vi "BinSearchVIHotwarm.vi"(8 "X0":sgl=0.5, 11 "Ring":i16(ring) items=["Warm", "Cold"]) -> (3 "Xpot":sgl)   [LabVIEW 2019]
uses:
  <vilib>/Platform/TimedLoop/XDataNode/timing_clust.ctl
  <vilib>/Platform/TimedLoop/XDataNode/nitl_modes.ctl
  <vilib>/Platform/TimedLoop/XDataNode/wakeup.ctl
  <vilib>/rvi/Emulation/niFpgaGetClockAttributes.vi
  <vilib>/rvi/Emulation/niFpgaSctlEmulationGetInTimedLoop.vi
  <vilib>/rvi/Emulation/niFpgaEmulationReportErrorSimple.vi
  <vilib>/rvi/Emulation/niFpgaCriticalErrorInLSC.vi
  <vilib>/Platform/TimedLoop/XDataNode/XDataNode.xnode
  <vilib>/Platform/TimedLoop/XDataNode/XDNodeRunTimeDep.lvlib
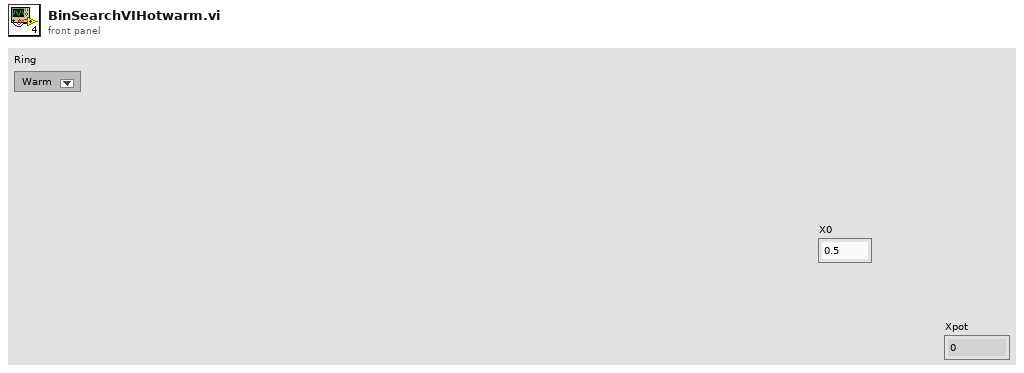
[diagram p1: front panel]
types:
  T1 = typedef "XDNodeRunTimeDep.lvlib/timing_clust.ctl" = cluster{"Expected End [f-1]":u64, "Actual End [f-1]":u64, "Finished Late? [f-1]":bool, "Expected End [i-1]":u64, "Actual End [i-1]":u64, "Finished Late? [i-1]":bool, "Expected Start [i]":u64, "Actual Start [i]":u64, "Expected Start [f]":u64, "Actual Start [f]":u64, "Source Name":string, "Structure Name":string, "Period":i64, "Deadline":i64, "Offset":i64, "Start":i64, "Priority":i32, "Timeout":i32, "Mode":T2, "Wakeup Reason":T3, "Error":errorcluster, "Source Type":string, "Secondary Source Type":string, "Global End Time":u64, "Global Start Time":u64, "Frame Duration":u64, "Iteration Duration":u64, "Assigned CPU":i32, "I/O Scan Engine Mode":u32}
  T2 = typedef "XDNodeRunTimeDep.lvlib/nitl_modes.ctl" = enum32{"No Change", "Process missed periods, maintain original phase", "Discard missed periods, maintain original phase", "Process missed periods, ignore original phase", "Discard missed periods, ignore original phase"}
  T3 = typedef "XDNodeRunTimeDep.lvlib/wakeup.ctl" = enum32{"Normal", "Aborted", "Asynchronous wakeup", "Timing source error", "Timed loop error", "Timeout"}
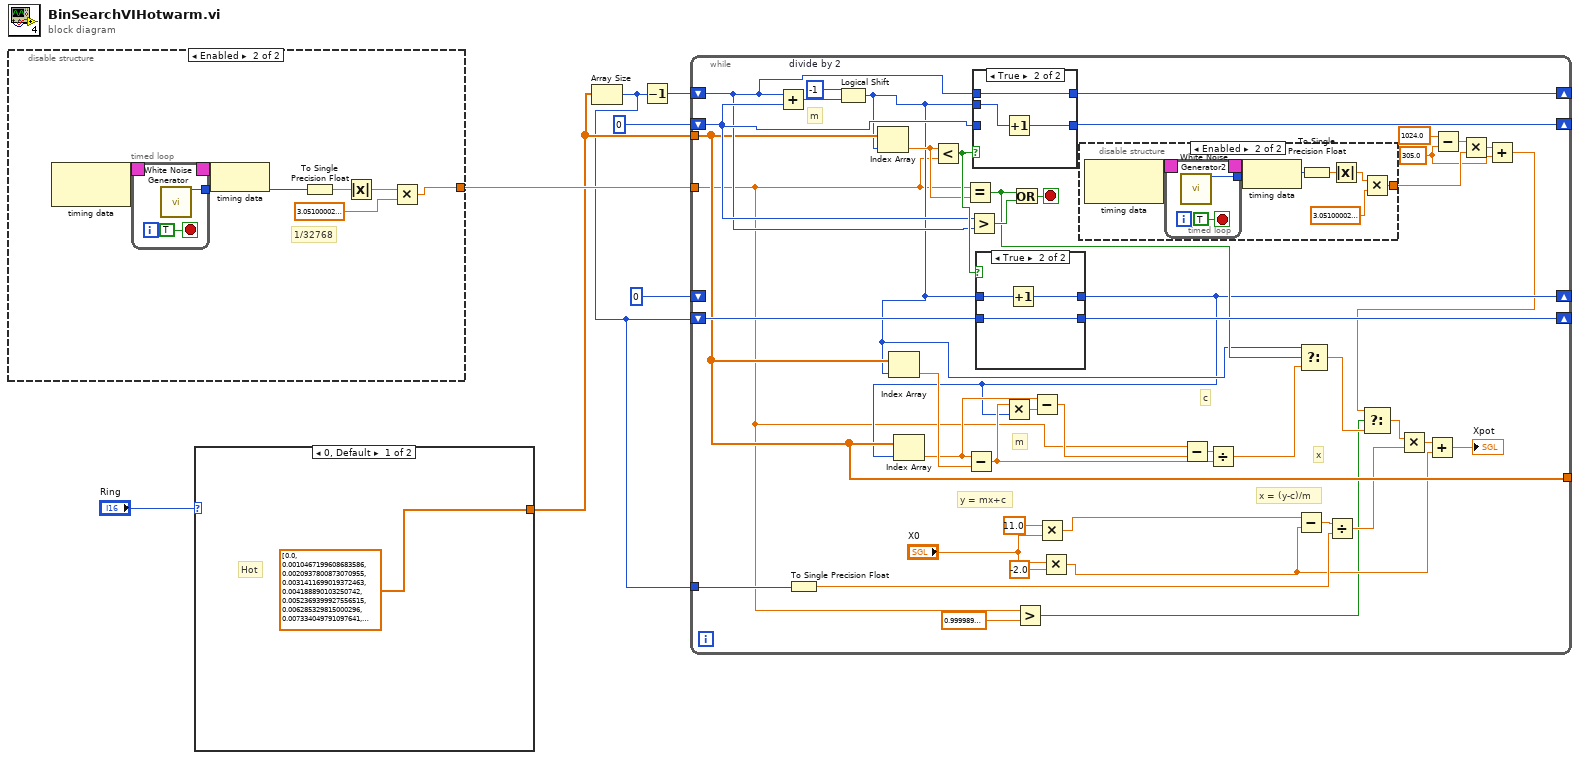
[diagram p0: block diagram]
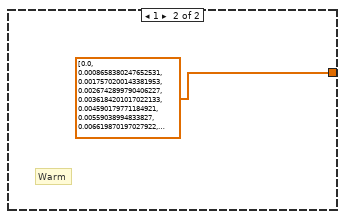
[diagram p2: hidden frame]
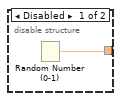
[diagram p3: hidden frame]
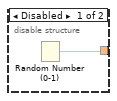
[diagram p4: hidden frame]
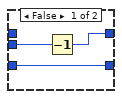
[diagram p6: hidden frame]
diagram:
  n1 = disable-structure shown="Enabled" {
    disable-tunnel: [w8 w11] -> w4
    frame Disabled {
      n2 = Random Number (0-1)() -> (number: 0 to 1=w8:dbl)
    }
    frame Enabled {
      # "1/32768"
      n3 = node-c288() -> (w10:T1)  [unwired: 1 in]
      n4 = timed-loop {
        timing: w10 -> [_]
        timing-out: [_] -> w9
        tunnel: [w17] -> w15
        stop <- TRUE stop-if-true
        n5 = call "White Noise Generator"() -> ("white noise out"=w17:i16)  [unwired: 15 in]
      }
      n6 = node-c288(w9) -> ()
      n7 = To Single Precision Float(number=w15) -> (single precision float=w13:sgl)
      n8 = Absolute Value(x=w13) -> (abs(x)=w12:sgl)
      n9 = Multiply(x=w12, y=sgl 3.051e-05) -> (x*y=w11:sgl)
    }
  }
  n10 = case shown="0, Default" "Ring" {
    tunnel: [sgl[] [0.0, 0.00104672, 0.00209378, 0.00314117, 0.00418889, 0.00523694, 0.00628533, 0.00733405, 0.0083831, 0.00943249, 0.0104822, 0.0115323, 0.0125826, 0.0136334, 0.0146844, 0.0157358, 0.0167875, 0.0178396, 0.018892, 0.0199447, 0.0209977, 0.0220511, 0.0231048, 0.0241589, 0.0252133, 0.026268, 0.0273231, 0.0283785, 0.0294342, 0.0304902, 0.0315466, 0.0326032, 0.0336601, 0.0347173, 0.0357748, 0.0368325, 0.0378905, 0.0389487, 0.0400072, 0.0410658, 0.0421247, 0.0431839, 0.0442432, 0.0453027, 0.0463624, 0.0474222, 0.0484823, 0.0495425, 0.0506029, 0.0516634, 0.0527241, 0.0537849, 0.0548458, 0.0559069, 0.0569681, 0.0580294, 0.0590909, 0.0601524, 0.061214, 0.0622757, 0.0633376, 0.0643995, 0.0654614, 0.0665235, 0.0675856, 0.0686478, 0.0697101, 0.0707724, 0.0718348, 0.0728972, 0.0739596, 0.0750221, 0.0760847, 0.0771473, 0.0782099, 0.0792725, 0.0803352, 0.0813978, 0.0824605, 0.0835233, 0.084586, 0.0856487, 0.0867115, 0.0877742, 0.088837, 0.0898997, 0.0909625, 0.0920252, 0.093088, 0.0941507, 0.0952134, 0.0962761, 0.0973388, 0.0984015, 0.0994642, 0.100527, 0.10159, 0.102652, 0.103715, 0.104777, 0.10584, 0.106902, 0.107965, 0.109027, 0.11009, 0.111152, 0.112215, 0.113277, 0.114339, 0.115402, 0.116464, 0.117526, 0.118589, 0.119651, 0.120713, 0.121775, 0.122837, 0.123899, 0.124961, 0.126023, 0.127085, 0.128147, 0.129209, 0.130271, 0.131333, 0.132395, 0.133457, 0.134519, 0.135581, 0.136642, 0.137704, 0.138766, 0.139828, 0.140889, 0.141951, 0.143013, 0.144075, 0.145136, 0.146198, 0.14726, 0.148321, 0.149383, 0.150444, 0.151506, 0.152568, 0.153629, 0.154691, 0.155752, 0.156814, 0.157876, 0.158937, 0.159999, 0.16106, 0.162122, 0.163184, 0.164245, 0.165307, 0.166368, 0.16743, 0.168492, 0.169553, 0.170615, 0.171677, 0.172739, 0.1738, 0.174862, 0.175924, 0.176986, 0.178048, 0.17911, 0.180171, 0.181233, 0.182295, 0.183357, 0.184419, 0.185482, 0.186544, 0.187606, 0.188668, 0.18973, 0.190792, 0.191855, 0.192917, 0.19398, 0.195042, 0.196104, 0.197167, 0.19823, 0.199292, 0.200355, 0.201418, 0.20248, 0.203543, 0.204606, 0.205669, 0.206732, 0.207795, 0.208858, 0.209921, 0.210985, 0.212048, 0.213111, 0.214174, 0.215238, 0.216301, 0.217365, 0.218428, 0.219492, 0.220556, 0.22162, 0.222683, 0.223747, 0.224811, 0.225875, 0.226939, 0.228003, 0.229067, 0.230131, 0.231196, 0.23226, 0.233324, 0.234389, 0.235453, 0.236517, 0.237582, 0.238646, 0.239711, 0.240776, 0.24184, 0.242905, 0.24397, 0.245034, 0.246099, 0.247164, 0.248229, 0.249293, 0.250358, 0.251423, 0.252488, 0.253553, 0.254618, 0.255683, 0.256747, 0.257812, 0.258877, 0.259942, 0.261007, 0.262072, 0.263136, 0.264201, 0.265266, 0.266331, 0.267395, 0.26846, 0.269525, 0.270589, 0.271654, 0.272718, 0.273782, 0.274847, 0.275911, 0.276975, 0.278039, 0.279103, 0.280167, 0.28123, 0.282294, 0.283357, 0.284421, 0.285484, 0.286547, 0.28761, 0.288673, 0.289735, 0.290798, 0.29186, 0.292922, 0.293984, 0.295046, 0.296107, 0.297169, 0.29823, 0.29929, 0.300351, 0.301411, 0.302471, 0.303531, 0.304591, 0.30565, 0.306709, 0.307768, 0.308826, 0.309884, 0.310942, 0.311999, 0.313056, 0.314112, 0.315169, 0.316225, 0.31728, 0.318336, 0.319391, 0.320445, 0.3215, 0.322554, 0.323607, 0.32466, 0.325713, 0.326766, 0.327818, 0.32887, 0.329922, 0.330973, 0.332024, 0.333075, 0.334125, 0.335175, 0.336225, 0.337274, 0.338323, 0.339372, 0.34042, 0.341468, 0.342515, 0.343563, 0.34461, 0.345656, 0.346703, 0.347749, 0.348794, 0.34984, 0.350884, 0.351929, 0.352973, 0.354017, 0.355061, 0.356104, 0.357147, 0.35819, 0.359232, 0.360274, 0.361316, 0.362357, 0.363398, 0.364439, 0.365479, 0.366519, 0.367559, 0.368598, 0.369637, 0.370676, 0.371714, 0.372752, 0.37379, 0.374828, 0.375865, 0.376901, 0.377938, 0.378974, 0.380009, 0.381045, 0.38208, 0.383115, 0.384149, 0.385183, 0.386217, 0.38725, 0.388283, 0.389316, 0.390349, 0.391381, 0.392412, 0.393444, 0.394475, 0.395506, 0.396536, 0.397566, 0.398596, 0.399626, 0.400655, 0.401684, 0.402712, 0.40374, 0.404768, 0.405796, 0.406823, 0.40785, 0.408877, 0.409903, 0.410929, 0.411954, 0.41298, 0.414005, 0.415029, 0.416053, 0.417077, 0.418101, 0.419124, 0.420147, 0.42117, 0.422192, 0.423214, 0.424236, 0.425257, 0.426278, 0.427299, 0.428319, 0.42934, 0.430359, 0.431379, 0.432398, 0.433417, 0.434435, 0.435453, 0.436471, 0.437488, 0.438506, 0.439522, 0.440539, 0.441555, 0.442571, 0.443586, 0.444602, 0.445617, 0.446631, 0.447645, 0.448659, 0.449673, 0.450686, 0.451699, 0.452712, 0.453724, 0.454736, 0.455748, 0.456759, 0.45777, 0.458781, 0.459791, 0.460802, 0.461811, 0.462821, 0.46383, 0.464839, 0.465847, 0.466855, 0.467863, 0.468871, 0.469878, 0.470885, 0.471891, 0.472897, 0.473903, 0.474909, 0.475914, 0.476919, 0.477924, 0.478928, 0.479932, 0.480936, 0.481939, 0.482942, 0.483945, 0.484947, 0.48595, 0.486951, 0.487953, 0.488954, 0.489955, 0.490955, 0.491955, 0.492955, 0.493955, 0.494954, 0.495953, 0.496952, 0.49795, 0.498948, 0.499946, 0.500943, 0.50194, 0.502937, 0.503933, 0.504929, 0.505925, 0.50692, 0.507915, 0.50891, 0.509905, 0.510899, 0.511893, 0.512886, 0.51388, 0.514872, 0.515865, 0.516857, 0.517849, 0.518841, 0.519832, 0.520823, 0.521814, 0.522804, 0.523794, 0.524784, 0.525774, 0.526763, 0.527752, 0.52874, 0.529728, 0.530716, 0.531704, 0.532691, 0.533678, 0.534665, 0.535651, 0.536637, 0.537623, 0.538608, 0.539593, 0.540578, 0.541562, 0.542546, 0.54353, 0.544514, 0.545497, 0.54648, 0.547462, 0.548445, 0.549427, 0.550408, 0.55139, 0.552371, 0.553351, 0.554332, 0.555312, 0.556291, 0.557271, 0.55825, 0.559229, 0.560207, 0.561186, 0.562164, 0.563141, 0.564118, 0.565095, 0.566072, 0.567048, 0.568024, 0.569, 0.569976, 0.570951, 0.571926, 0.5729, 0.573874, 0.574848, 0.575822, 0.576795, 0.577768, 0.57874, 0.579713, 0.580685, 0.581657, 0.582628, 0.583599, 0.58457, 0.58554, 0.586511, 0.58748, 0.58845, 0.589419, 0.590388, 0.591357, 0.592325, 0.593293, 0.594261, 0.595228, 0.596195, 0.597162, 0.598129, 0.599095, 0.600061, 0.601026, 0.601992, 0.602957, 0.603921, 0.604886, 0.60585, 0.606813, 0.607777, 0.60874, 0.609703, 0.610665, 0.611627, 0.612589, 0.613551, 0.614512, 0.615473, 0.616434, 0.617394, 0.618354, 0.619314, 0.620273, 0.621233, 0.622191, 0.62315, 0.624108, 0.625066, 0.626024, 0.626981, 0.627938, 0.628895, 0.629851, 0.630807, 0.631763, 0.632719, 0.633674, 0.634629, 0.635583, 0.636538, 0.637492, 0.638445, 0.639399, 0.640352, 0.641305, 0.642257, 0.643209, 0.644161, 0.645113, 0.646064, 0.647015, 0.647966, 0.648916, 0.649866, 0.650816, 0.651765, 0.652714, 0.653663, 0.654612, 0.65556, 0.656508, 0.657456, 0.658403, 0.65935, 0.660297, 0.661243, 0.662189, 0.663135, 0.664081, 0.665026, 0.665971, 0.666916, 0.66786, 0.668804, 0.669748, 0.670691, 0.671635, 0.672577, 0.67352, 0.674462, 0.675404, 0.676346, 0.677287, 0.678228, 0.679169, 0.680109, 0.681049, 0.681989, 0.682929, 0.683868, 0.684807, 0.685746, 0.686684, 0.687622, 0.68856, 0.689497, 0.690435, 0.691371, 0.692308, 0.693244, 0.69418, 0.695116, 0.696051, 0.696986, 0.697921, 0.698856, 0.69979, 0.700724, 0.701657, 0.702591, 0.703524, 0.704457, 0.705389, 0.706321, 0.707253, 0.708185, 0.709116, 0.710047, 0.710978, 0.711908, 0.712838, 0.713768, 0.714697, 0.715626, 0.716555, 0.717484, 0.718412, 0.71934, 0.720268, 0.721195, 0.722122, 0.723049, 0.723976, 0.724902, 0.725828, 0.726754, 0.727679, 0.728604, 0.729529, 0.730453, 0.731378, 0.732301, 0.733225, 0.734148, 0.735071, 0.735994, 0.736917, 0.737839, 0.738761, 0.739682, 0.740603, 0.741524, 0.742445, 0.743365, 0.744285, 0.745205, 0.746125, 0.747044, 0.747963, 0.748882, 0.7498, 0.750718, 0.751636, 0.752553, 0.75347, 0.754387, 0.755304, 0.75622, 0.757136, 0.758052, 0.758967, 0.759882, 0.760797, 0.761712, 0.762626, 0.76354, 0.764454, 0.765367, 0.76628, 0.767193, 0.768106, 0.769018, 0.76993, 0.770841, 0.771753, 0.772664, 0.773575, 0.774485, 0.775395, 0.776305, 0.777215, 0.778124, 0.779033, 0.779942, 0.780851, 0.781759, 0.782667, 0.783574, 0.784482, 0.785389, 0.786296, 0.787202, 0.788108, 0.789014, 0.78992, 0.790825, 0.79173, 0.792635, 0.793539, 0.794443, 0.795347, 0.796251, 0.797154, 0.798057, 0.79896, 0.799862, 0.800765, 0.801666, 0.802568, 0.803469, 0.80437, 0.805271, 0.806172, 0.807072, 0.807972, 0.808871, 0.809771, 0.81067, 0.811568, 0.812467, 0.813365, 0.814263, 0.81516, 0.816058, 0.816955, 0.817851, 0.818748, 0.819644, 0.82054, 0.821436, 0.822331, 0.823226, 0.824121, 0.825015, 0.825909, 0.826803, 0.827697, 0.82859, 0.829483, 0.830376, 0.831268, 0.832161, 0.833053, 0.833944, 0.834835, 0.835727, 0.836617, 0.837508, 0.838398, 0.839288, 0.840178, 0.841067, 0.841956, 0.842845, 0.843733, 0.844622, 0.84551, 0.846397, 0.847285, 0.848172, 0.849059, 0.849945, 0.850831, 0.851717, 0.852603, 0.853489, 0.854374, 0.855259, 0.856143, 0.857027, 0.857911, 0.858795, 0.859679, 0.860562, 0.861445, 0.862327, 0.86321, 0.864092, 0.864974, 0.865855, 0.866736, 0.867617, 0.868498, 0.869378, 0.870258, 0.871138, 0.872018, 0.872897, 0.873776, 0.874655, 0.875533, 0.876411, 0.877289, 0.878167, 0.879044, 0.879921, 0.880798, 0.881674, 0.882551, 0.883427, 0.884302, 0.885178, 0.886053, 0.886927, 0.887802, 0.888676, 0.88955, 0.890424, 0.891297, 0.892171, 0.893043, 0.893916, 0.894788, 0.89566, 0.896532, 0.897404, 0.898275, 0.899146, 0.900016, 0.900887, 0.901757, 0.902627, 0.903496, 0.904366, 0.905235, 0.906103, 0.906972, 0.90784, 0.908708, 0.909575, 0.910443, 0.91131, 0.912177, 0.913043, 0.913909, 0.914775, 0.915641, 0.916506, 0.917372, 0.918236, 0.919101, 0.919965, 0.920829, 0.921693, 0.922557, 0.92342, 0.924283, 0.925146, 0.926008, 0.92687, 0.927732, 0.928594, 0.929455, 0.930316, 0.931177, 0.932037, 0.932897, 0.933757, 0.934617, 0.935476, 0.936336, 0.937194, 0.938053, 0.938911, 0.939769, 0.940627, 0.941485, 0.942342, 0.943199, 0.944055, 0.944912, 0.945768, 0.946624, 0.947479, 0.948335, 0.94919, 0.950045, 0.950899, 0.951753, 0.952607, 0.953461, 0.954314, 0.955168, 0.95602, 0.956873, 0.957725, 0.958577, 0.959429, 0.960281, 0.961132, 0.961983, 0.962834, 0.963684, 0.964534, 0.965384, 0.966234, 0.967083, 0.967932, 0.968781, 0.96963, 0.970478, 0.971326, 0.972174, 0.973021, 0.973869, 0.974715, 0.975562, 0.976409, 0.977255, 0.978101, 0.978946, 0.979791, 0.980637, 0.981481, 0.982326, 0.98317, 0.984014, 0.984858, 0.985701, 0.986544, 0.987387, 0.98823, 0.989072, 0.989914, 0.990756, 0.991598, 0.992439, 0.99328, 0.994121, 0.994962, 0.995802, 0.996642, 0.997482, 0.998321, 0.99916, 0.999999] ("Init Data Out") sgl[] [0.0, 0.000865838, 0.00175702, 0.00267429, 0.00361842, 0.00459018, 0.00559039, 0.00661987, 0.0076795, 0.00877014, 0.00989271, 0.0110481, 0.0122374, 0.0134615, 0.0147214, 0.0160181, 0.0173529, 0.0187267, 0.0201407, 0.0215961, 0.0230942, 0.0246361, 0.0262231, 0.0278565, 0.0295378, 0.0312683, 0.0330498, 0.0348832, 0.0367683, 0.0387052, 0.0406935, 0.0427329, 0.044823, 0.0469636, 0.0491541, 0.0513939, 0.0536825, 0.0560193, 0.0584036, 0.0608346, 0.0633115, 0.0658336, 0.0683999, 0.0710095, 0.0736616, 0.076355, 0.0790889, 0.0818621, 0.0846736, 0.0875224, 0.0904072, 0.0933269, 0.0962805, 0.0992667, 0.102284, 0.105332, 0.108409, 0.111514, 0.114646, 0.117803, 0.120985, 0.12419, 0.127416, 0.130664, 0.133931, 0.137217, 0.14052, 0.143839, 0.147174, 0.150523, 0.153884, 0.157258, 0.160643, 0.164038, 0.167441, 0.170853, 0.174272, 0.177698, 0.181129, 0.184564, 0.188003, 0.191445, 0.19489, 0.198336, 0.201783, 0.20523, 0.208676, 0.212122, 0.215565, 0.219007, 0.222446, 0.225881, 0.229313, 0.232741, 0.236164, 0.239582, 0.242995, 0.246402, 0.249804, 0.253199, 0.256587, 0.259969, 0.263344, 0.266712, 0.270072, 0.273425, 0.276771, 0.280108, 0.283438, 0.286761, 0.290075, 0.293381, 0.29668, 0.29997, 0.303253, 0.306527, 0.309795, 0.313054, 0.316306, 0.31955, 0.322787, 0.326016, 0.329239, 0.332454, 0.335663, 0.338865, 0.34206, 0.34525, 0.348433, 0.351611, 0.354783, 0.35795, 0.361111, 0.364268, 0.36742, 0.370568, 0.373713, 0.376853, 0.37999, 0.383123, 0.386254, 0.389383, 0.392509, 0.395634, 0.398756, 0.401878, 0.404999, 0.408119, 0.411239, 0.414359, 0.41748, 0.420602, 0.423725, 0.426849, 0.429976, 0.433104, 0.436236, 0.43937, 0.442508, 0.44565, 0.448796, 0.451946, 0.455101, 0.458262, 0.461428, 0.4646, 0.467779, 0.470964, 0.474157, 0.477357, 0.480565, 0.483782, 0.487007, 0.490241, 0.493484, 0.496738, 0.500001, 0.503275, 0.506559, 0.509855, 0.513162, 0.516481, 0.519812, 0.523156, 0.526513, 0.529882, 0.533265, 0.536662, 0.540073, 0.543498, 0.546938, 0.550393, 0.553862, 0.557348, 0.560848, 0.564365, 0.567898, 0.571446, 0.575012, 0.578594, 0.582192, 0.585808, 0.58944, 0.59309, 0.596757, 0.600441, 0.604143, 0.607862, 0.611598, 0.615352, 0.619123, 0.622911, 0.626717, 0.630539, 0.634379, 0.638235, 0.642109, 0.645998, 0.649904, 0.653825, 0.657762, 0.661715, 0.665682, 0.669664, 0.67366, 0.67767, 0.681692, 0.685727, 0.689775, 0.693833, 0.697902, 0.701981, 0.70607, 0.710167, 0.714272, 0.718383, 0.722501, 0.726624, 0.73075, 0.73488, 0.739012, 0.743145, 0.747277, 0.751408, 0.755537, 0.759661, 0.763781, 0.767894, 0.772, 0.776096, 0.780182, 0.784256, 0.788316, 0.792362, 0.79639, 0.800401, 0.804392, 0.808362, 0.812309, 0.816232, 0.820128, 0.823996, 0.827836, 0.831643, 0.835419, 0.839159, 0.842864, 0.846531, 0.850159, 0.853745, 0.857289, 0.860789, 0.864243, 0.86765, 0.871009, 0.874317, 0.877573, 0.880777, 0.883927, 0.887021, 0.890059, 0.893039, 0.89596, 0.898821, 0.901622, 0.904361, 0.907038, 0.909651, 0.912201, 0.914687, 0.917108, 0.919465, 0.921755, 0.92398, 0.926142, 0.928243, 0.930284, 0.932267, 0.934193, 0.936065, 0.937883, 0.93965, 0.941366, 0.943034, 0.944654, 0.946228, 0.947757, 0.949243, 0.950687, 0.952089, 0.953452, 0.954776, 0.956062, 0.957312, 0.958526, 0.959705, 0.960851, 0.961965, 0.963047, 0.964098, 0.965119, 0.966111, 0.967075, 0.968011, 0.968921, 0.969805, 0.970664, 0.971498, 0.972309, 0.973096, 0.973861, 0.974605, 0.975327, 0.976029, 0.976711, 0.977373, 0.978016, 0.978642, 0.979249, 0.979839, 0.980413, 0.98097, 0.981511, 0.982037, 0.982548, 0.983044, 0.983527, 0.983995, 0.98445, 0.984893, 0.985322, 0.98574, 0.986145, 0.986539, 0.986922, 0.987294, 0.987656, 0.988007, 0.988348, 0.988679, 0.989001, 0.989314, 0.989618, 0.989913, 0.9902, 0.990479, 0.99075, 0.991013, 0.991268, 0.991517, 0.991758, 0.991992, 0.99222, 0.992441, 0.992656, 0.992865, 0.993068, 0.993265, 0.993457, 0.993643, 0.993824, 0.993999, 0.99417, 0.994336, 0.994497, 0.994654, 0.994806, 0.994953, 0.995097, 0.995236, 0.995372, 0.995504, 0.995631, 0.995756, 0.995876, 0.995994, 0.996108, 0.996218, 0.996326, 0.996431, 0.996532, 0.996631, 0.996727, 0.99682, 0.99691, 0.996998, 0.997083, 0.997166, 0.997247, 0.997325, 0.997401, 0.997475, 0.997547, 0.997617, 0.997685, 0.997751, 0.997815, 0.997877, 0.997937, 0.997996, 0.998053, 0.998108, 0.998162, 0.998214, 0.998265, 0.998314, 0.998362, 0.998409, 0.998454, 0.998498, 0.998541, 0.998583, 0.998623, 0.998662, 0.9987, 0.998737, 0.998773, 0.998808, 0.998842, 0.998875, 0.998907, 0.998938, 0.998968, 0.998998, 0.999026, 0.999054, 0.999081, 0.999107, 0.999132, 0.999157, 0.999181, 0.999204, 0.999227, 0.999249, 0.99927, 0.999291, 0.999311, 0.999331, 0.99935, 0.999369, 0.999387, 0.999404, 0.999421, 0.999438, 0.999454, 0.999469, 0.999484, 0.999499, 0.999513, 0.999527, 0.999541, 0.999554, 0.999566, 0.999579, 0.999591, 0.999602, 0.999614, 0.999625, 0.999635, 0.999646, 0.999656, 0.999666, 0.999675, 0.999684, 0.999693, 0.999702, 0.999711, 0.999719, 0.999727, 0.999735, 0.999742, 0.99975, 0.999757, 0.999764, 0.99977, 0.999777, 0.999783, 0.999789, 0.999795, 0.999801, 0.999807, 0.999812, 0.999818, 0.999823, 0.999828, 0.999833, 0.999838, 0.999842, 0.999847, 0.999851, 0.999856, 0.99986, 0.999864, 0.999867, 0.999871, 0.999875, 0.999879, 0.999882, 0.999885, 0.999889, 0.999892, 0.999895, 0.999898, 0.999901, 0.999904, 0.999906, 0.999909, 0.999912, 0.999914, 0.999917, 0.999919, 0.999921, 0.999924, 0.999926, 0.999928, 0.99993, 0.999932, 0.999934, 0.999936, 0.999938, 0.99994, 0.999941, 0.999943, 0.999945, 0.999946, 0.999948, 0.999949, 0.999951, 0.999952, 0.999954, 0.999955, 0.999956, 0.999958, 0.999959, 0.99996, 0.999961, 0.999962, 0.999963, 0.999964, 0.999965, 0.999966, 0.999967, 0.999968, 0.999969, 0.99997, 0.999971, 0.999972, 0.999973, 0.999973, 0.999974, 0.999975, 0.999976, 0.999976, 0.999977, 0.999978, 0.999978, 0.999979, 0.99998, 0.99998, 0.999981, 0.999981, 0.999982, 0.999983, 0.999983, 0.999984, 0.999984, 0.999985, 0.999985, 0.999985, 0.999986, 0.999986, 0.999987, 0.999987, 0.999988, 0.999988, 0.999988, 0.999989, 0.999989, 0.999989, 0.99999, 0.99999, 0.99999, 0.999991, 0.999991, 0.999991, 0.999991, 0.999992, 0.999992, 0.999992, 0.999992, 0.999993, 0.999993, 0.999993, 0.999993, 0.999994, 0.999994, 0.999994, 0.999994, 0.999994, 0.999994, 0.999995, 0.999995, 0.999995, 0.999995, 0.999995, 0.999996, 0.999996, 0.999996, 0.999996, 0.999996, 0.999996, 0.999996, 0.999996, 0.999997, 0.999997, 0.999997, 0.999997, 0.999997, 0.999997, 0.999997, 0.999997, 0.999997, 0.999998, 0.999998, 0.999998, 0.999998, 0.999998, 0.999998, 0.999998, 0.999998, 0.999998, 0.999998, 0.999998, 0.999998, 0.999998, 0.999998, 0.999999, 0.999999, 0.999999, 0.999999, 0.999999, 0.999999, 0.999999, 0.999999, 0.999999, 0.999999, 0.999999, 0.999999, 0.999999, 0.999999, 0.999999, 0.999999, 0.999999, 1.0, 1.0, 1.0, 1.0, 1.0, 1.0, 1.0, 1.0, 1.0, 1.0, 1.0, 1.0, 1.0, 1.0, 1.0, 1.0, 1.0, 1.0, 1.0, 1.0, 1.0, 1.0, 1.0, 1.0, 1.0, 1.0, 1.0, 1.0, 1.0, 1.0, 1.0, 1.0, 1.0, 1.0, 1.0, 1.0, 1.0, 1.0, 1.0, 1.0, 1.0, 1.0, 1.0, 1.0, 1.0, 1.0, 1.0, 1.0, 1.0, 1.0, 1.0, 1.0, 1.0, 1.0, 1.0, 1.0, 1.0, 1.0, 1.0, 1.0, 1.0, 1.0, 1.0, 1.0, 1.0, 1.0, 1.0, 1.0, 1.0, 1.0, 1.0, 1.0, 1.0, 1.0, 1.0, 1.0, 1.0, 1.0, 1.0, 1.0, 1.0, 1.0, 1.0, 1.0, 1.0, 1.0, 1.0, 1.0, 1.0, 1.0, 1.0, 1.0, 1.0, 1.0, 1.0, 1.0, 1.0, 1.0, 1.0, 1.0, 1.0, 1.0, 1.0, 1.0, 1.0, 1.0, 1.0, 1.0, 1.0, 1.0, 1.0, 1.0, 1.0, 1.0, 1.0, 1.0, 1.0, 1.0, 1.0, 1.0, 1.0, 1.0, 1.0, 1.0, 1.0, 1.0, 1.0, 1.0, 1.0, 1.0, 1.0, 1.0, 1.0, 1.0, 1.0, 1.0, 1.0, 1.0, 1.0, 1.0, 1.0, 1.0, 1.0, 1.0, 1.0, 1.0, 1.0, 1.0, 1.0, 1.0, 1.0, 1.0, 1.0, 1.0, 1.0, 1.0, 1.0, 1.0, 1.0, 1.0, 1.0, 1.0, 1.0, 1.0, 1.0, 1.0, 1.0, 1.0, 1.0, 1.0, 1.0, 1.0, 1.0, 1.0, 1.0, 1.0, 1.0, 1.0, 1.0, 1.0, 1.0, 1.0, 1.0, 1.0, 1.0, 1.0, 1.0, 1.0, 1.0, 1.0, 1.0, 1.0, 1.0, 1.0, 1.0, 1.0, 1.0, 1.0, 1.0, 1.0, 1.0, 1.0, 1.0, 1.0, 1.0, 1.0, 1.0, 1.0, 1.0, 1.0, 1.0, 1.0, 1.0, 1.0, 1.0, 1.0, 1.0, 1.0, 1.0, 1.0, 1.0, 1.0, 1.0, 1.0, 1.0, 1.0, 1.0, 1.0, 1.0, 1.0, 1.0, 1.0, 1.0, 1.0, 1.0, 1.0, 1.0, 1.0, 1.0, 1.0, 1.0, 1.0, 1.0, 1.0, 1.0, 1.0, 1.0, 1.0, 1.0, 1.0, 1.0, 1.0, 1.0, 1.0, 1.0, 1.0, 1.0, 1.0, 1.0, 1.0, 1.0, 1.0, 1.0, 1.0, 1.0, 1.0, 1.0, 1.0, 1.0, 1.0, 1.0, 1.0, 1.0, 1.0, 1.0, 1.0, 1.0, 1.0, 1.0, 1.0, 1.0, 1.0, 1.0, 1.0, 1.0, 1.0, 1.0, 1.0, 1.0, 1.0, 1.0, 1.0, 1.0, 1.0, 1.0, 1.0, 1.0, 1.0, 1.0, 1.0, 1.0, 1.0, 1.0, 1.0, 1.0, 1.0, 1.0, 1.0, 1.0, 1.0, 1.0, 1.0, 1.0, 1.0, 1.0, 1.0, 1.0, 1.0, 1.0, 1.0, 1.0, 1.0, 1.0, 1.0, 1.0, 1.0, 1.0, 1.0, 1.0, 1.0, 1.0, 1.0, 1.0, 1.0, 1.0, 1.0, 1.0, 1.0, 1.0, 1.0, 1.0, 1.0, 1.0, 1.0, 1.0, 1.0, 1.0, 1.0, 1.0, 1.0, 1.0] ("Init Data Out")] -> w2
    frame 0, Default {
      # "Hot"
    }
    frame 1 {
      # "Warm"
    }
  }
  n11 = Array Size(array=w2) -> (size(s)=w1:i32)
  n12 = Decrement(x=w1) -> (x-1=w5:i32)
  n13 = while {
    tunnel: w2 -> [w55]
    tunnel: w4 -> [w34]
    shift-right: [w67] -> _
    shift-left: w5 -> [w58]
    shift-right: [w63] -> _
    shift-left: 0 -> [w59]
    shift-right: [w46] -> _
    shift-left: 0 -> [_]
    shift-right: [w60] -> _
    shift-left: w1 -> [w61]
    tunnel: [w55] -> _
    tunnel: w1 -> [w40]
    stop <- w65 stop-if-true
    w27 = sgl 305.0 ("y")
    w68 = -1  # divide by 2
    # "x"
    # "x = (y-c)/m"
    # "c"
    # "m"
    # "y = mx+c"
    # "m"
    n14 = Add(x=w58, y=w59) -> (x+y=w64:i32)
    n15 = To Single Precision Float(number=w40) -> (single precision float=w39:sgl)
    n16 = Logical Shift(y=w68, x=w64) -> (x << y=w53:i32)
    n17 = Index Array(array=w55, index=w53) -> (element=w57:sgl)
    n18 = Index Array(array=w55, index=w53) -> (element=w56:sgl)
    n19 = Less?(x=w57, y=w34) -> (x < y?=w62:bool)
    n20 = Equal?(x=w34, y=w57) -> (x = y?=w54:bool)
    n21 = Greater?(x=w59, y=w58) -> (0:w66:bool)
    n22 = case shown="True" w62 {
      tunnel: w53 -> [w90 w93]
      tunnel: [w89 w91] -> w67
      tunnel: w59 -> [w88 _]
      tunnel: [w88 w92] -> w63
      tunnel: w58 -> [_ w91]
      frame False {
        n23 = Decrement(x=w90) -> (x-1=w89:i32)
      }
      frame True {
        n24 = Increment(x=w93) -> (x+1=w92:i32)
      }
    }
    n25 = case shown="True" w62 {
      tunnel: w53 -> [w84 w87]
      tunnel: [w83 w86] -> w46
      tunnel: w61 -> [w83 w85]
      tunnel: [w84 w85] -> w60
      frame False {
      }
      frame True {
        n26 = Increment(x=w87) -> (x+1=w86:i32)
      }
    }
    n27 = Index Array(array=w55, index=w46) -> (element=w51:sgl)
    n28 = Subtract(x=w51, y=w56) -> (x-y=w48:sgl)
    n29 = Multiply(x=w48, y=w46) -> (x*y=w52:sgl)
    n30 = Or(x=w54, y=w66) -> (x .or. y?=w65:bool)
    n31 = Greater?(x=w34, y=sgl 0.99999) -> (0:w24:bool)
    n32 = Subtract(x=w51, y=w52) -> (x-y=w50:sgl)
    n33 = Multiply(x=sgl 11.0, y="X0") -> (x*y=w43:sgl)
    n34 = Multiply(x="X0", y=sgl -2.0) -> (x*y=w37:sgl)
    n35 = disable-structure shown="Enabled" {
      disable-tunnel: [w69 w72] -> w29
      frame Disabled {
        n36 = Random Number (0-1)() -> (number: 0 to 1=w69:dbl)
      }
      frame Enabled {
        n37 = node-c288() -> (w71:T1)  [unwired: 1 in]
        n38 = timed-loop {
          timing: w71 -> [_]
          timing-out: [_] -> w70
          tunnel: [w78] -> w76
          stop <- TRUE stop-if-true
          n39 = call "White Noise Generator2"() -> ("white noise out"=w78:i16)  [unwired: 15 in]
        }
        n40 = node-c288(w70) -> ()
        n41 = To Single Precision Float(number=w76) -> (single precision float=w74:sgl)
        n42 = Absolute Value(x=w74) -> (abs(x)=w73:sgl)
        n43 = Multiply(x=w73, y=sgl 3.051e-05) -> (x*y=w72:sgl)
      }
    }
    n44 = Subtract(x=w34, y=w50) -> (x-y=w49:sgl)
    n45 = Divide(x=w49, y=w48) -> (x/y=w47:sgl)
    n46 = Subtract(x=w43, y=w37) -> (x-y=w42:sgl)
    n47 = Select(t=w53, s=w54, f=w47) -> (s? t:f=w32:sgl)
    n48 = Divide(x=w42, y=w39) -> (x/y=w41:sgl)
    n49 = Subtract(x=sgl 1024.0, y=w27) -> (x-y=w30:sgl)
    n50 = Multiply(x=w30, y=w29) -> (x*y=w28:sgl)
    n51 = Add(x=w28, y=w27) -> (x+y=w25:sgl)
    n52 = Select(t=w25, s=w24, f=w32) -> (s? t:f=w26:sgl)
    n53 = Multiply(x=w26, y=w41) -> (x*y=w38:sgl)
    n54 = Add(x=w38, y=w37) -> (x+y=→"Xpot":sgl)
  }
